vi "FGV Stoerungen sammeln und auswerten.vi"(0 "Errors":T1, 2 "Neustart":bool, 3 "Abbrechen":bool, 4 "Fortsetzen":bool, 5 "error in (no error)":errorcluster caption="Fehler (Eingang, kein Fehler)", 6 "keep Errors for AutoSPAN":bool, 11 "Aktion":T2) -> (12 "Errors for AutoSPAN":T1, 14 "Errors":T1, 15 "Error":bool, 16 "Neustart":bool, 17 "Abbrechen":bool, 18 "Fortsetzen":bool, 19 "error out":errorcluster caption="Fehler (Ausgang)")   [LabVIEW 2020, in "Linearisierung v2.lvlib"]
uses:
  Linearisierung v2.lvlib
  Aktion FGV Stoerungen sammeln und auswerten.ctl
  LIN ErrorCluster.ctl
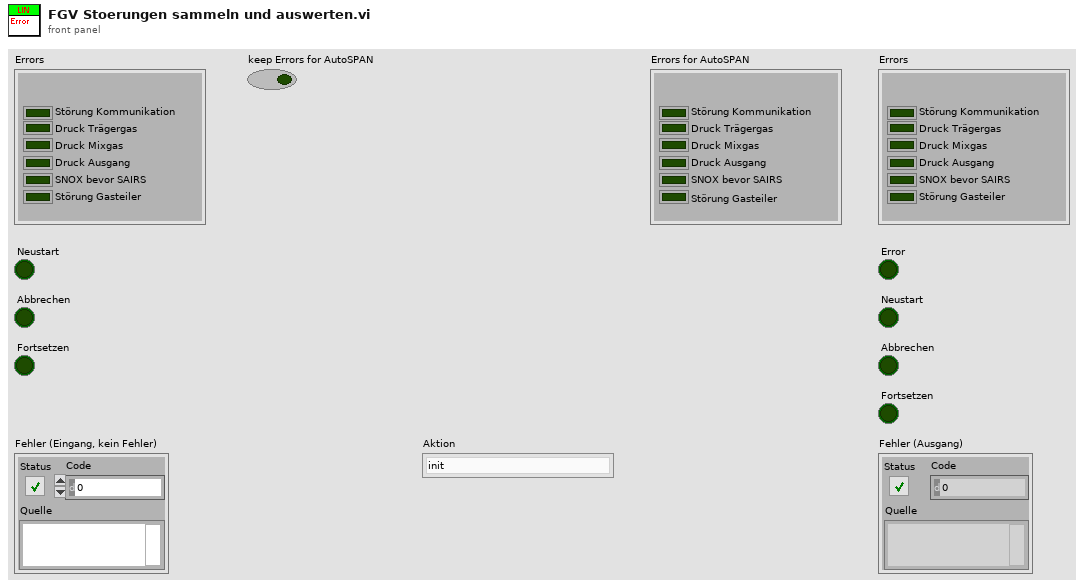
[diagram p1: front panel]
types:
  T1 = typedef "Linearisierung v2.lvlib/LIN ErrorCluster.ctl" = cluster{"Störung Kommunikation":bool, "Pressure carrier gas":bool, "Pressure diluted gas":bool, "Outlet Pressure":bool, "SNOX before SAIR":bool, "Störung Gasteiler":bool}
  T2 = typedef "Linearisierung v2.lvlib/Aktion FGV Stoerungen sammeln und auswerten.ctl" = enum16{"init", "lesen", "error", "prüfen", "reset error", "abbrechen", "fortsetzen", "neustart", "Bedientasten reset"}
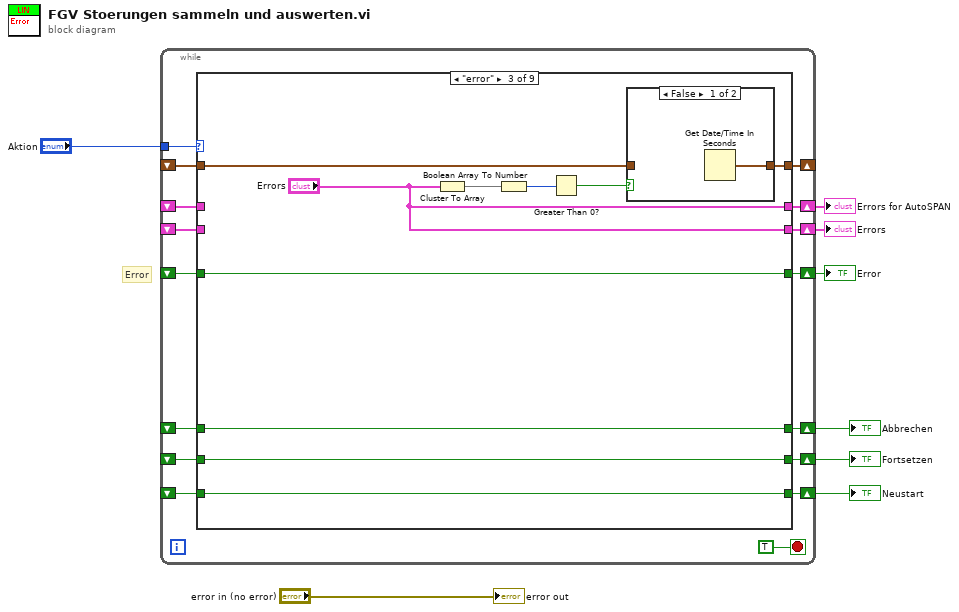
[diagram p0: block diagram]
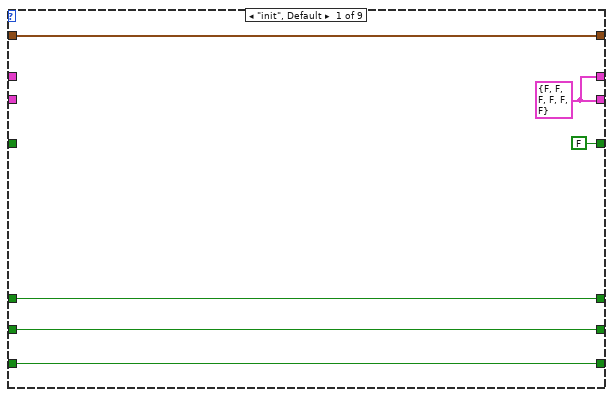
[diagram p2: hidden frame]
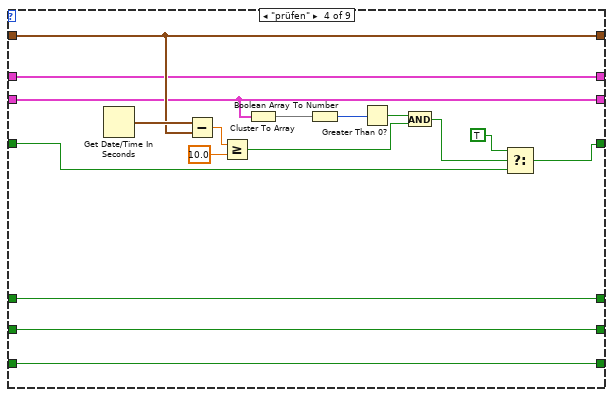
[diagram p5: hidden frame]
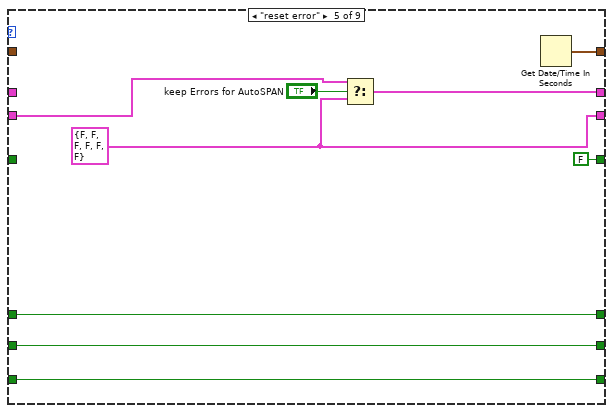
[diagram p6: hidden frame]
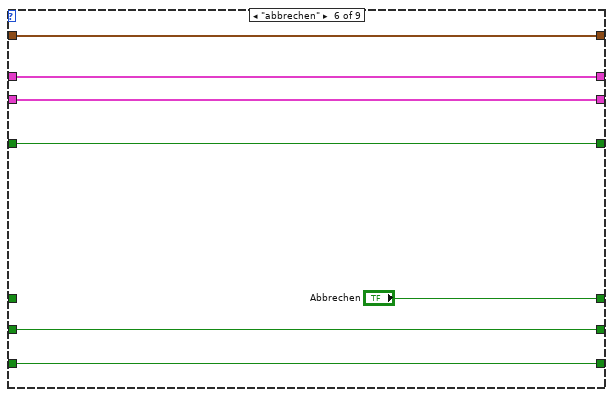
[diagram p7: hidden frame]
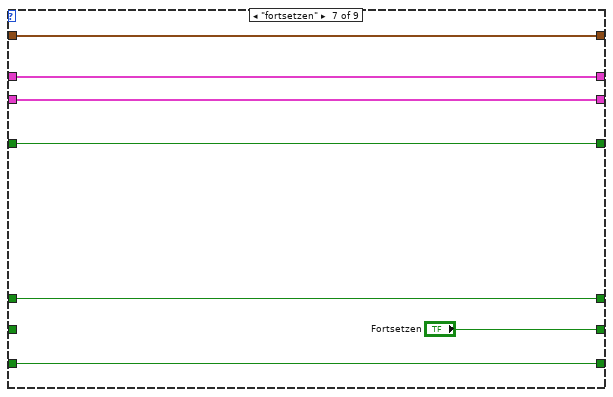
[diagram p8: hidden frame]
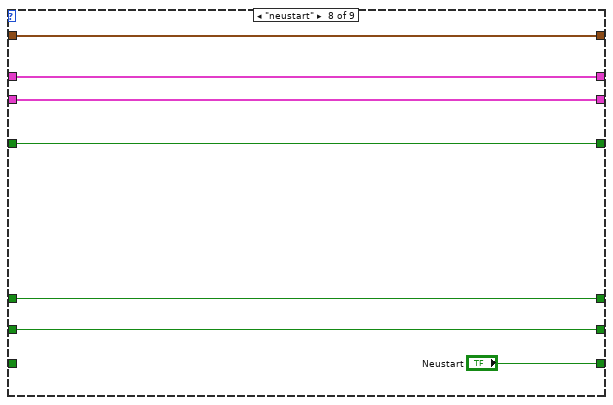
[diagram p9: hidden frame]
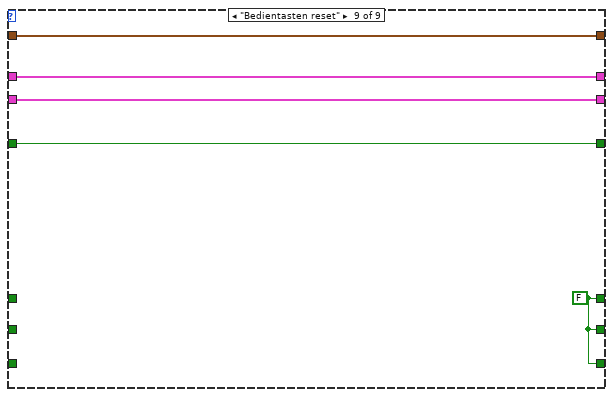
[diagram p10: hidden frame]
diagram:
  # "Error"
  n1 = while {
    tunnel: "Aktion" -> [w23]
    shift-right: [w22] -> _
    shift-left: _ -> [w21]
    shift-right: [w20] -> w7
    shift-left: _ -> [w19]
    shift-right: [w18] -> w6
    shift-left: _ -> [w17]
    shift-right: [w16] -> w5
    shift-left: _ -> [w15]
    shift-right: [w14] -> w3
    shift-left: _ -> [w13]
    shift-right: [w12] -> w4
    shift-left: _ -> [w11]
    shift-right: [w10] -> w2
    shift-left: _ -> [w9]
    stop <- TRUE stop-if-true
    n2 = case shown="\"error\"" w23 {
      tunnel: [w29 w37 w45 w65 w71 w82 w89 w96 w101] -> w22
      tunnel: w21 -> [w29 w37 w44 w65 _ w82 w89 w96 w101]
      tunnel: [FALSE w36 w43 w54 FALSE ("x UND y?") w81 w88 w95 w100] -> w20
      tunnel: w19 -> [_ w36 w43 w55 _ w81 w88 w95 w100]
      tunnel: [w25 w35 "Errors" w59 w68 w80 w87 w94 w99] -> w18
      tunnel: w17 -> [_ w35 _ w59 w69 w80 w87 w94 w99]
      tunnel: [w28 w34 w41 w53 w74 "Abbrechen" w86 w93 w98] -> w16
      tunnel: w15 -> [w28 w34 w41 w53 w74 _ w86 w93 _]
      tunnel: [w27 w33 w40 w52 w73 w78 "Fortsetzen" w92 w98] -> w14
      tunnel: w13 -> [w27 w33 w40 w52 w73 w78 _ w92 _]
      tunnel: [w26 w32 w39 w51 w72 w77 w84 "Neustart" w98] -> w12
      tunnel: w11 -> [w26 w32 w39 w51 w72 w77 w84 _ _]
      tunnel: [w25 w31 "Errors" w50 w67 w76 w83 w90 w97] -> w10
      tunnel: w9 -> [_ w31 _ w50 _ w76 w83 w90 w97]
      frame "init", Default {
        w25 = T1 {"Störung Kommunikation"=FALSE, "Pressure carrier gas"=FALSE, "Pressure diluted gas"=FALSE, "Outlet Pressure"=FALSE, "SNOX before SAIR"=FALSE, "Störung Gasteiler"=FALSE} ("Errors")
      }
      frame "lesen" {
      }
      frame "error" {
        n3 = Cluster To Array(cluster="Errors") -> (array=w47:bool[])
        n4 = Boolean Array To Number(Boolean array=w47) -> (number=w46:u32)
        n5 = Greater Than 0?(x=w46) -> (x > 0?=w42:bool)
        n6 = case shown="False" w42 {
          tunnel: [w48 w49] -> w45
          tunnel: w44 -> [_ w49]
          frame False {
            n7 = Get Date/Time In Seconds() -> (seconds since 1Jan1904=w48:timestamp)
          }
          frame True {
          }
        }
      }
      frame "prüfen" {
        n8 = Get Date/Time In Seconds() -> (seconds since 1Jan1904=w66:timestamp)
        n9 = Subtract(x=w66, y=w65) -> (x-y=w64:dbl)
        n10 = Greater Or Equal?(x=w64, y=10.0) -> (x >= y?=w62:bool)
        n11 = Cluster To Array(cluster=w59) -> (array=w61:bool[])
        n12 = Boolean Array To Number(Boolean array=w61) -> (number=w60:u32)
        n13 = Greater Than 0?(x=w60) -> (x > 0?=w58:bool)
        n14 = And(x=w58, y=w62) -> (x .and. y?=w57:bool)
        n15 = Select(t=TRUE ("x UND y?"), s=w57, f=w55) -> (s? t:f=w54:bool)
      }
      frame "reset error" {
        w68 = T1 {"Störung Kommunikation"=FALSE, "Pressure carrier gas"=FALSE, "Pressure diluted gas"=FALSE, "Outlet Pressure"=FALSE, "SNOX before SAIR"=FALSE, "Störung Gasteiler"=FALSE} ("Errors")
        n16 = Select(t=w69, s="keep Errors for AutoSPAN", f=w68) -> (s? t:f=w67:T1)
        n17 = Get Date/Time In Seconds() -> (seconds since 1Jan1904=w71:timestamp)
      }
      frame "abbrechen" {
      }
      frame "fortsetzen" {
      }
      frame "neustart" {
      }
      frame "Bedientasten reset" {
        w98 = FALSE ("Abbrechen")
      }
    }
  }
  "Error" <- w7
  "Errors" <- w6
  "Abbrechen" <- w5
  "Fortsetzen" <- w3
  "Neustart" <- w4
  "Errors for AutoSPAN" <- w2
  "error out" <- "error in (no error)"
